vi "VecBuilder_2x1Fill.vi"(10 "R1":dbl, 11 "R0":dbl) -> (3 "output matrix":T1)   [LabVIEW 2019, in "Trajectory_Library.lvlib"]
doc: "Build a 2 x 1 Matrix (vector) from an array of input values.\n\nInputs:\n -- R0 -- Input value 1\n -- R1 -- Input value 2\n\nOutputs:\n -- Output Matrix -- Resulting 2 x 1 matrix (vector)"
uses:
  Trajectory_Library.lvlib
  <vilib>/Analysis/Matrix/Datatypes/RealMatrix.ctl
  <vilib>/Analysis/Matrix/NI_Matrix.lvlib
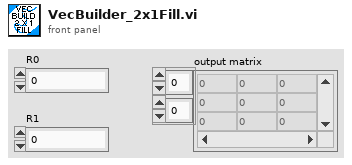
[diagram p1: front panel]
types:
  T1 = typedef "NI_Matrix.lvlib/RealMatrix.ctl" = dbl[][]
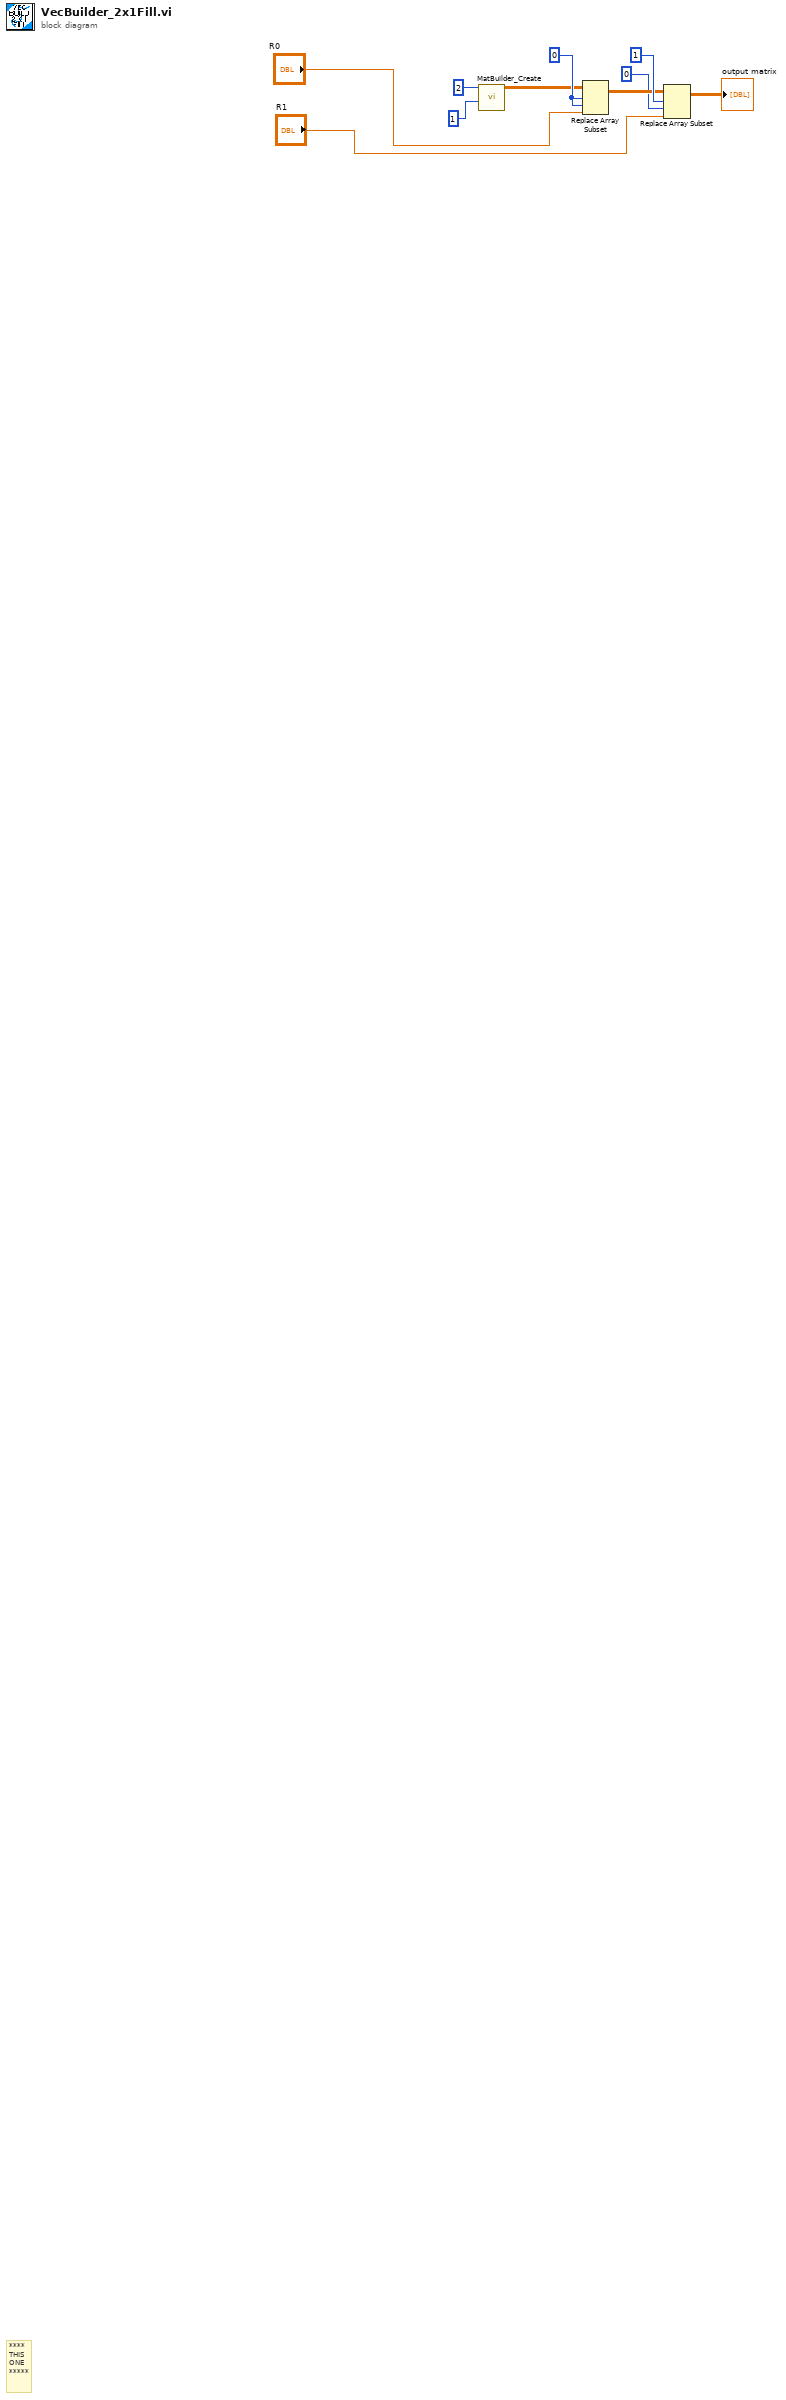
[diagram p0: block diagram]
diagram:
  w10 = 0 ("index (col)")
  # "****\nTHIS\nONE\n*****"
  n1 = call "MatBuilder_Create.vi"("Columns"=1, "Rows"=2) -> ("output matrix"=w1:T1)  [unwired: 9 in]
  n2 = Replace Array Subset(array=w1, new element="R0", index (row)=w10, index (col)=w10) -> (w8:T1)
  n3 = Replace Array Subset(array=w8, new element="R1", index (row)=1 ("index (col)"), index (col)=0 ("disabled index (col)")) -> (→"output matrix":T1)
